vi "Module_SP_GameDisplay.vi"(8 "error in (no error)":errorcluster, 9 "Module ID":i32=-1, 10 "Wait on Module(s) (\"\": none)":string) -> (0 "error out":errorcluster)   [LabVIEW 2019, in "Module_SP_GameDisplay.lvclass"]
doc: "JSMA Module Template - SubPanels 0.2.0.9\nRob Humfeld - Jet Engineering\nCopyright (c) 2019, Jet Engineering"
uses:
  Module_SP_GameDisplay.lvclass
  <userlib>/Jet Engineering/JSMA Signal Abstraction Layer (SAL)/CORE/jModule_SAL Class/jModule_SAL_ModuleType STYP.ctl
  Private/Module_SP_GameDisplay_RxMsg STYP.ctl
  <userlib>/Jet Engineering/JSMA/Libraries/jMsg_CORE/jMsg_JSMA_ApplicationShutdown/jMsg_JSMA_ApplicationShutdown.lvclass
  C:/Program Files/National Instruments/LabVIEW 2019/user.lib/Jet Engineering/JSMA/Libraries/jMsg Class/jMsg.lvclass
  Private/Module_SP_GameDisplay_TxMsg STYP.ctl
  C:/Program Files/National Instruments/LabVIEW 2019/user.lib/Jet Engineering/JSMA GUISubPanel CORE/jModule_GUISubPanel.lvclass
  C:/Program Files/National Instruments/LabVIEW 2019/user.lib/Jet Engineering/JSMA/Libraries/jModule Class/jModule.lvclass
  C:/Program Files/National Instruments/LabVIEW 2019/user.lib/JET Engineering/JSMA Signal Abstraction Layer (SAL)/CORE/jModule_SAL Class/jModule_SAL.lvclass
  Private/Module_SP_GameDisplay_Status STYP.ctl
  <userlib>/Jet Engineering/JSMA/Libraries/jModule Class/jModule.lvclass/jModule.ctl
  Module_SP_GameDisplay.lvclass/Module_SP_GameDisplay.ctl
  <userlib>/Jet Engineering/JET_QSM/Code/Private/JET_QSM - Add State [String API].vi
  <userlib>/Jet Engineering/JET_QSM/Code/Private/JET_QSM - Add State to Front [String API].vi
  <userlib>/Jet Engineering/JSMA/Libraries/jModule Class/jModule - Set Static Timer.vi
  <userlib>/Jet Engineering/JSMA/Libraries/jModule Class/jModule - Set Periodic Timer.vi
  <vilib>/Utility/error.llb/Trim Whitespace.vi
  <vilib>/Utility/error.llb/Error Cluster From Error Code.vi
  <userlib>/Jet Labs/JET Panel/JETPanel.lvclass
  <userlib>/Jet Engineering/JSMA/Libraries/jModule Class/jModule.lvclass
  <userlib>/JET Engineering/JSMA Signal Abstraction Layer (SAL)/CORE/jModule_SAL Class/jModule_SAL.lvclass
  <userlib>/Jet Engineering/JSMA GUISubPanel CORE/jModule_GUISubPanel.lvclass
  <userlib>/Jet Engineering/JSMA Signal Abstraction Layer (SAL)/CORE/SALSignal Class/SALSignal.lvclass
panel:
  out "jModule Name":string
  out "winSizer 2":string="W"
  out "winSizer 1":string="W"
  out "Recent states before Error (with tick counts)":string="0.167 sec ago: VI Initialize\n0.167 sec ago: Window Open\n0.110 sec ago: Control Update\n0.110 sec ago: Indicator Update\n0.000 sec ago: Error Handler\r\n"
  # "CENTER"
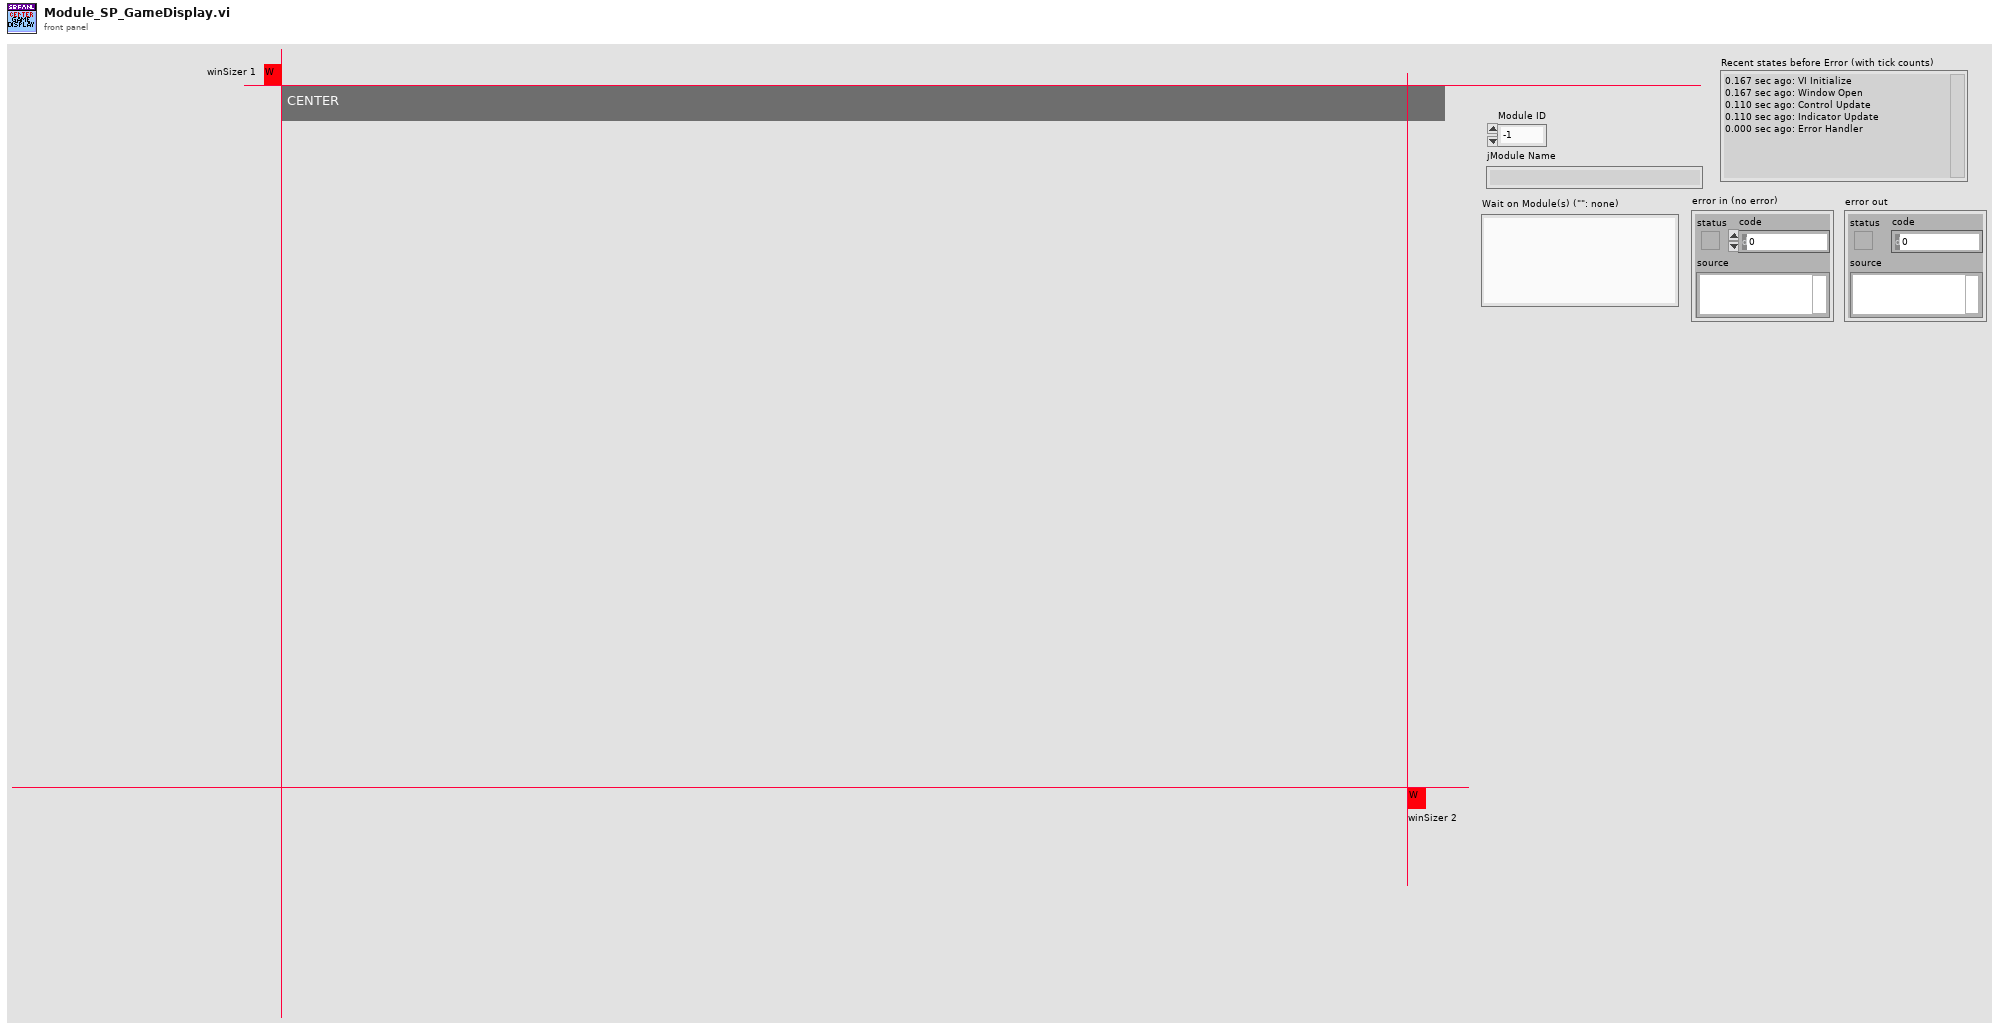
[diagram p1: front panel]
types:
  T1 = typedef "JSMA SAL CORE.lvlib/jModule_SAL.lvclass/jModule_SAL_ModuleType STYP.ctl" = enum16{"<no SAL functionality>", "Tag Data Client", "Tag Data Server", "Tag Data Server/Client"}
  T2 = typedef "Module_SP_GameDisplay.lvclass/Module_SP_GameDisplay_TxMsg STYP.ctl" = cluster{"<placeholder>":refnum<class "jMsg_JSMA_ApplicationShutdown.lvclass">}
  T3 = typedef "Module_SP_GameDisplay.lvclass/Module_SP_GameDisplay_RxMsg STYP.ctl" = cluster{"<placeholder>":refnum<class "jMsg_JSMA_ApplicationShutdown.lvclass">}
  T4 = typedef "Module_SP_GameDisplay.lvclass/Module_SP_GameDisplay_Status STYP.ctl" = cluster{"VI":cluster{"error":errorcluster, "isExiting?":bool}, "UI":cluster{"Placeholder":bool}}
  T5 = typedef "JET_QSM_Refnum STYP.ctl" = cluster{"state":cluster{"queue":refnum<queue>, "idle":string, "error":string, "STOP":string}, "debug":cluster{"enabled?":bool, "queue":refnum<queue>}, "Invalid.option":T6, "QSM.Name":string}
  T6 = typedef "JET_QSM_InvalidOption STYP.ctl" = enum16{"Ignore", "Dialog", "Error"}
  T7 = typedef "JET_QSM_Element STYP.ctl" = cluster{"state":string, "data":variant, "comment":string}
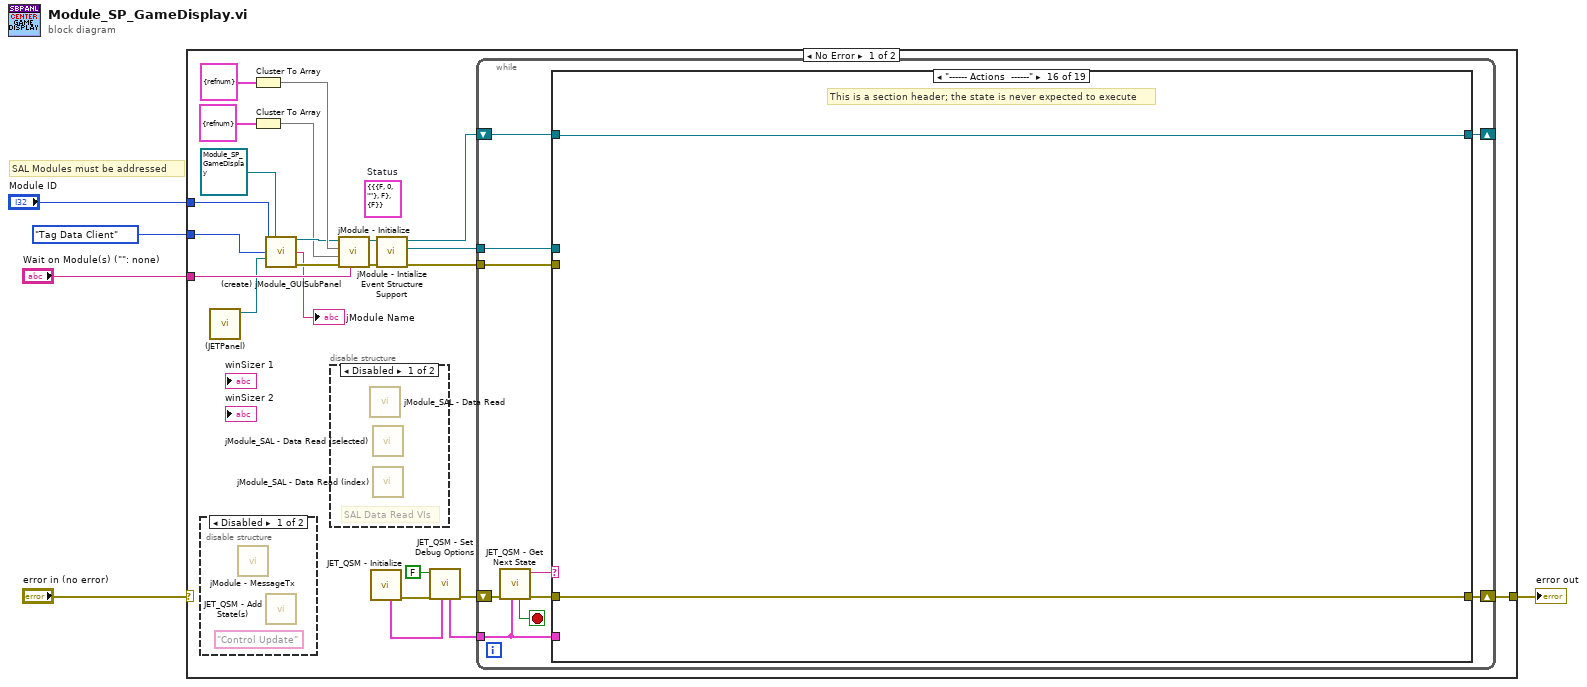
[diagram p0: block diagram]
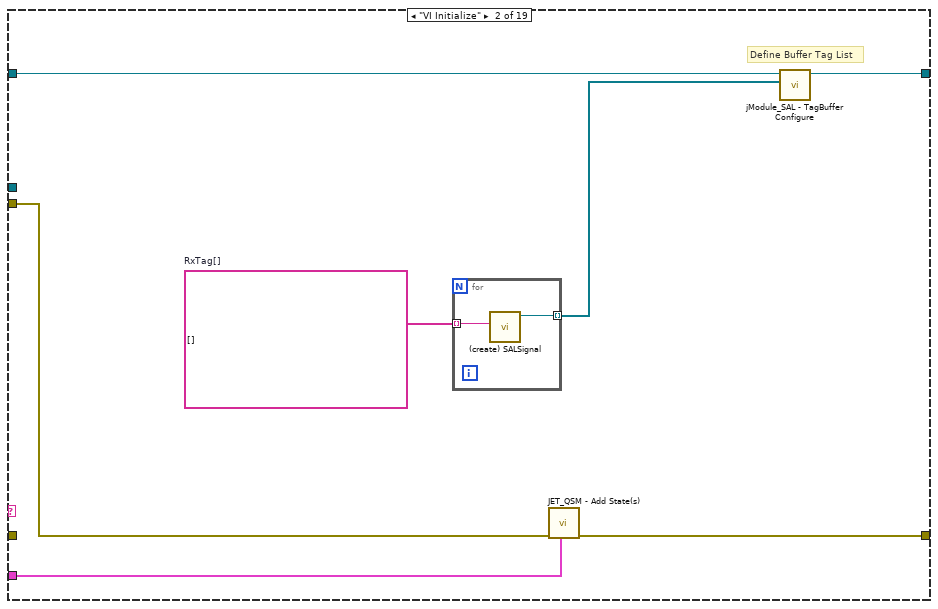
[diagram p5: hidden frame]
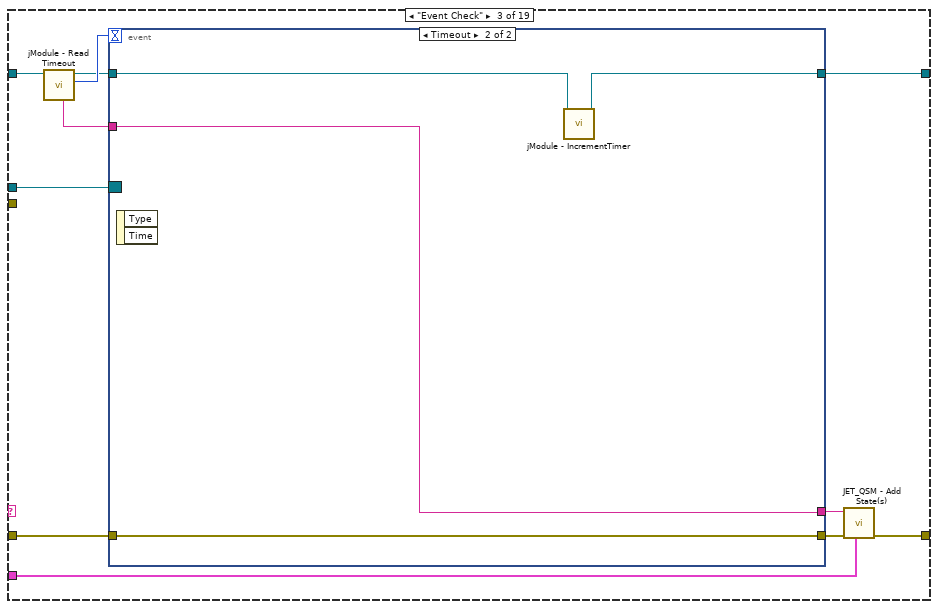
[diagram p6: hidden frame]
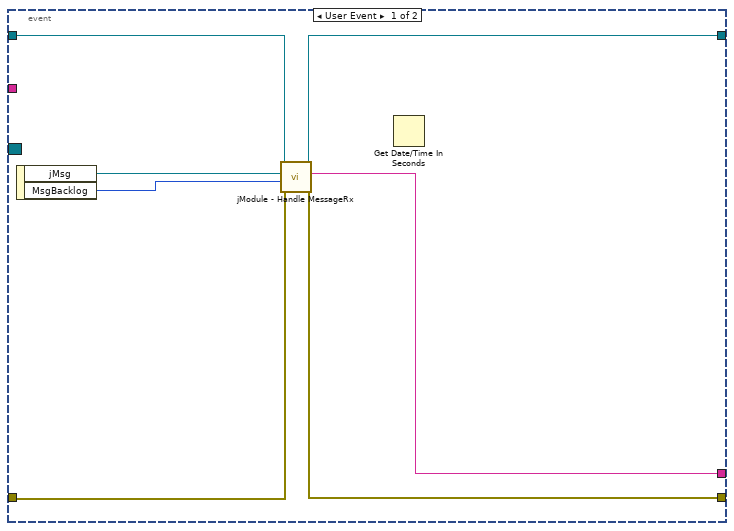
[diagram p7: hidden frame]
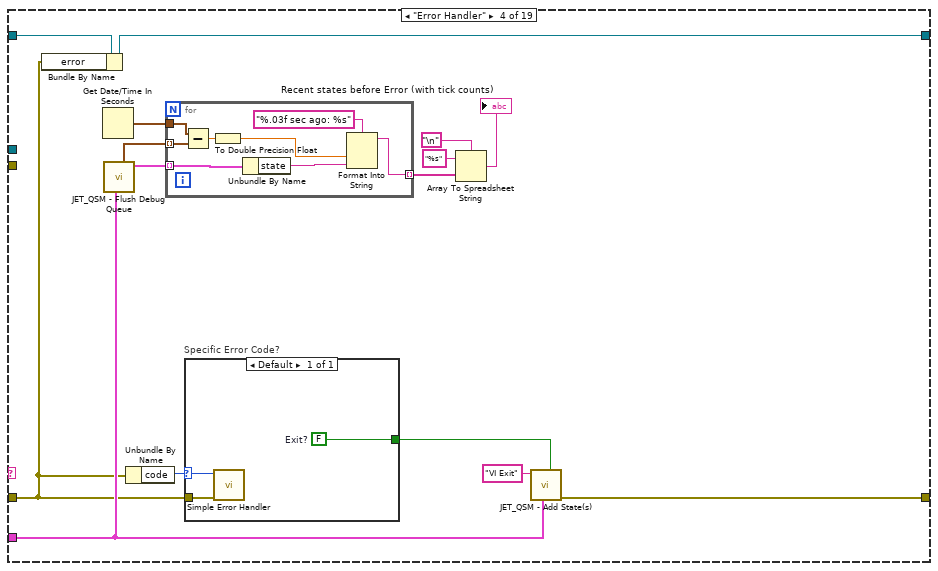
[diagram p8: hidden frame]
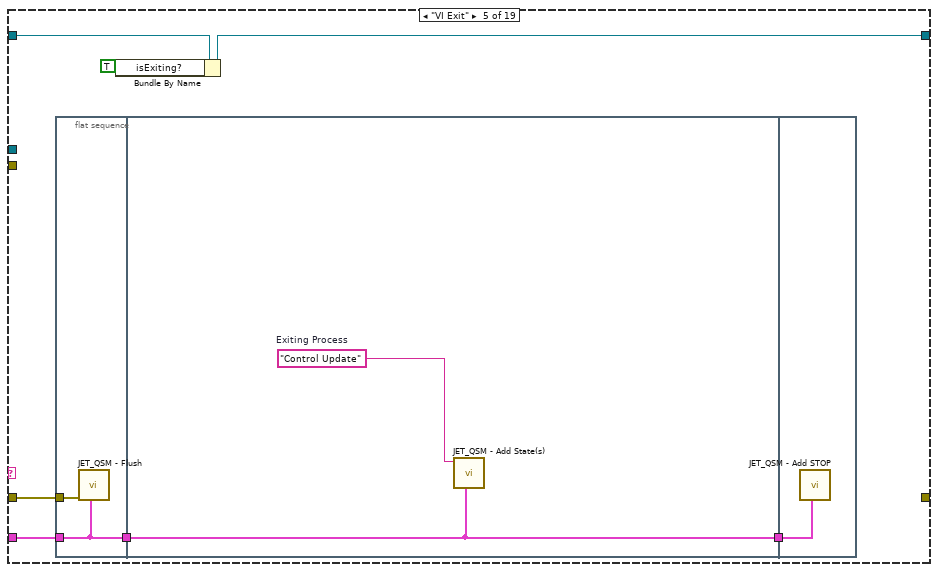
[diagram p9: hidden frame]
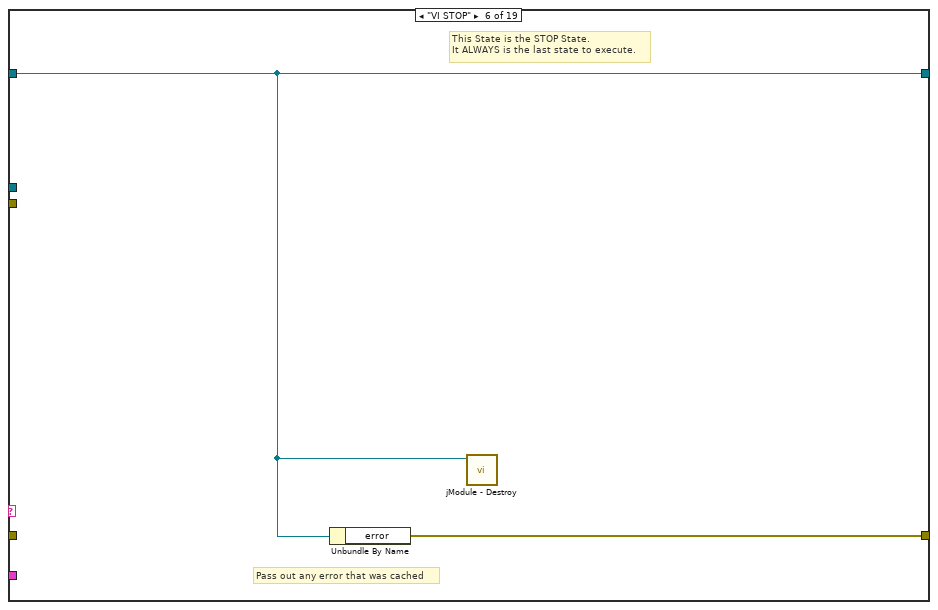
[diagram p10: hidden frame]
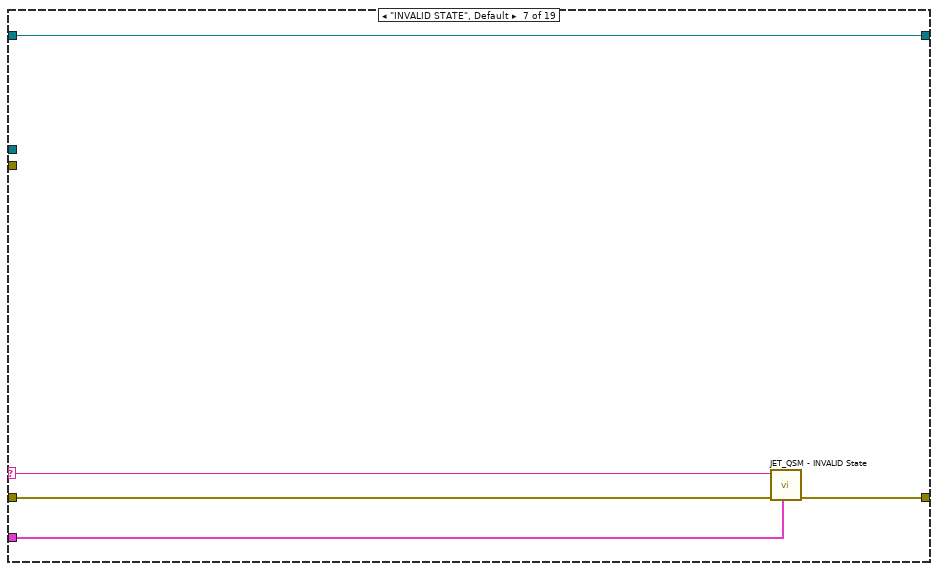
[diagram p11: hidden frame]
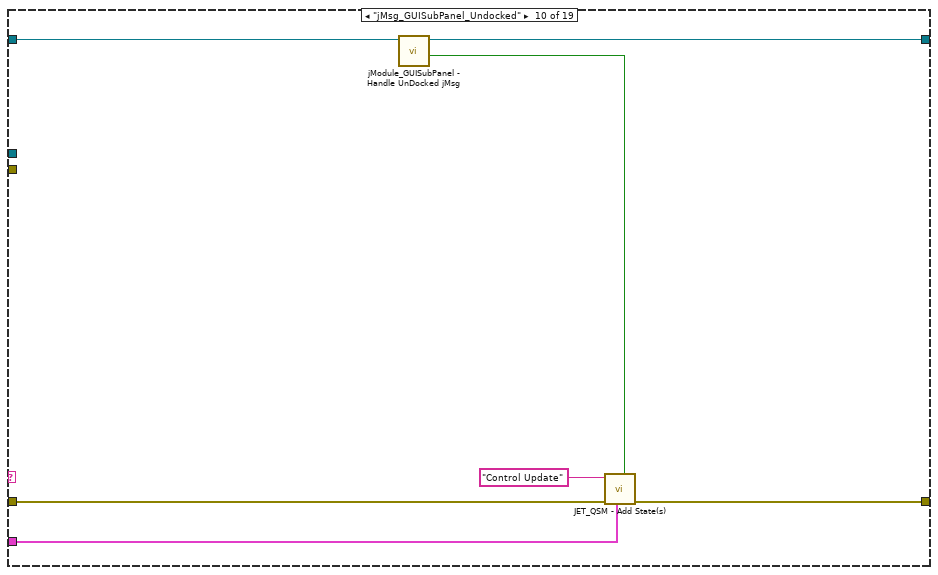
[diagram p14: hidden frame]
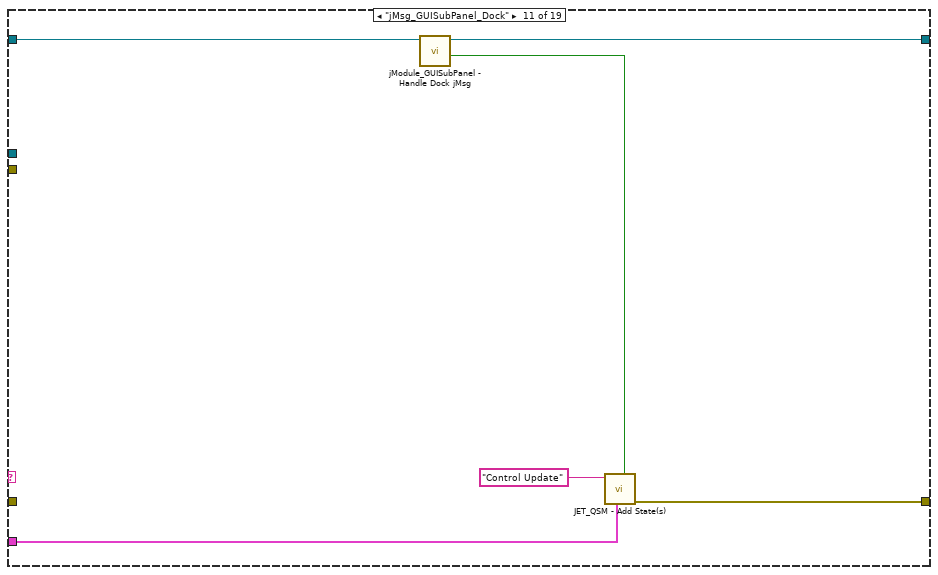
[diagram p15: hidden frame]
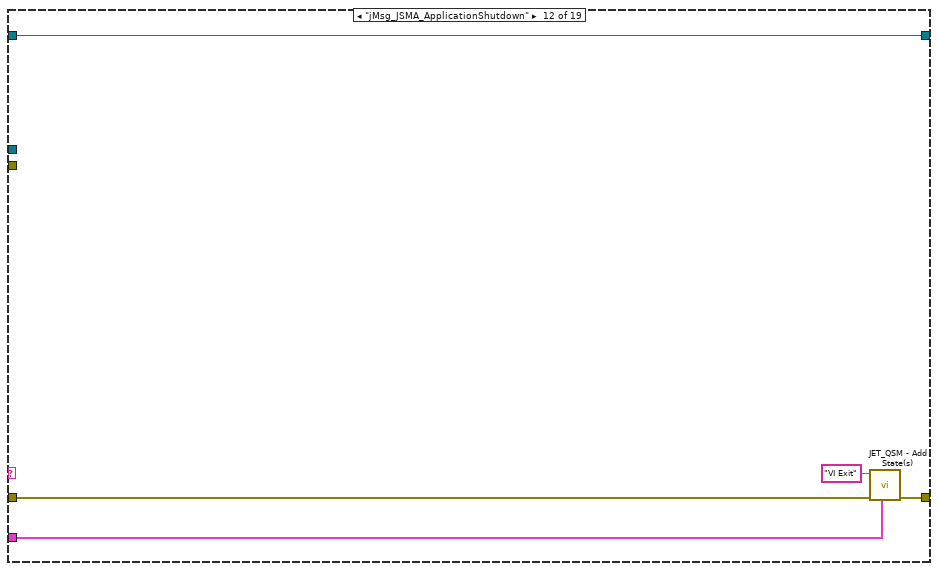
[diagram p16: hidden frame]
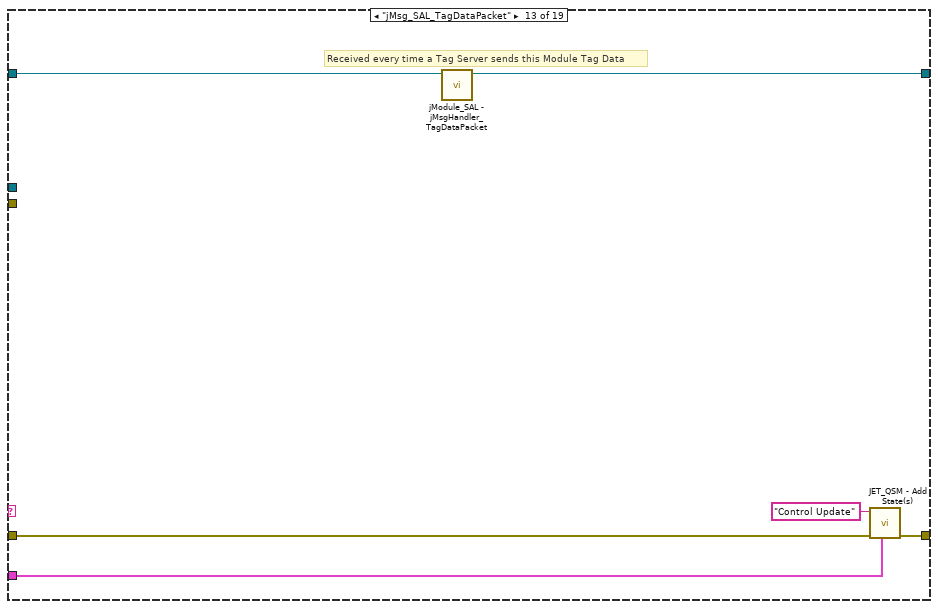
[diagram p17: hidden frame]
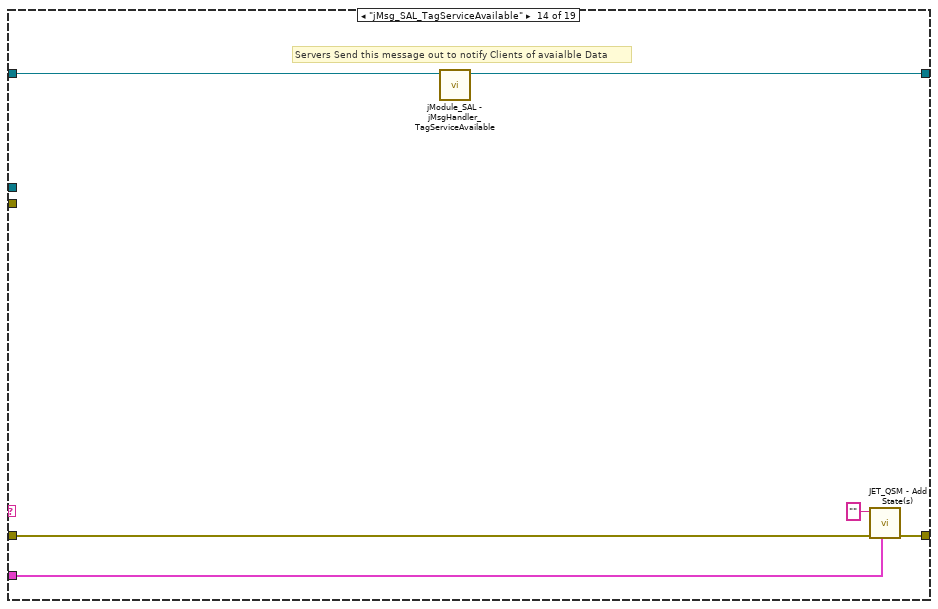
[diagram p18: hidden frame]
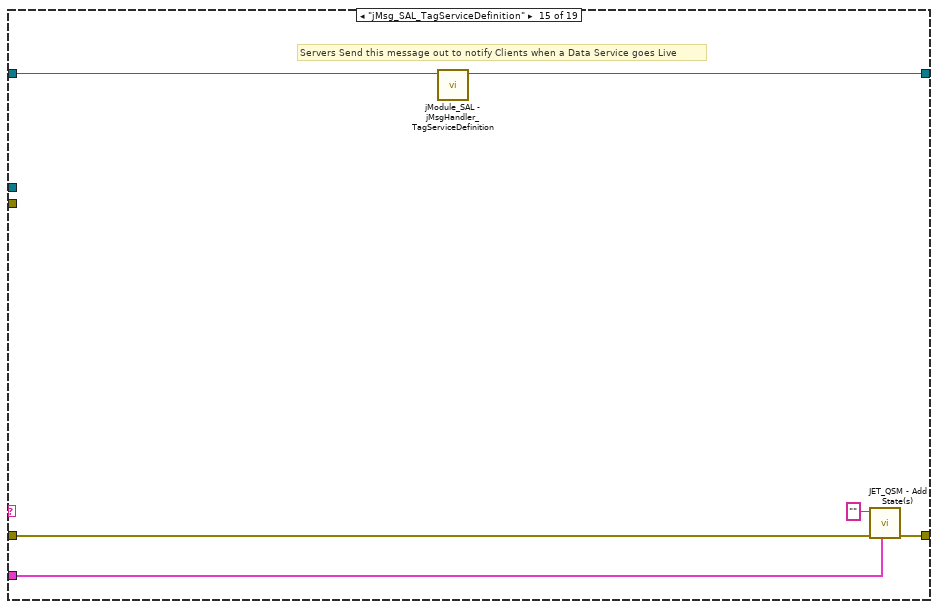
[diagram p19: hidden frame]
diagram:
  # "SAL Modules must be addressed"
  n1 = case shown="No Error" "error in (no error)" {
    selector: "error in (no error)" -> [_ w168]
    tunnel: [w28 w168] -> w5
    tunnel: "Wait on Module(s) (\"\": none)" -> [w17 _]
    tunnel: "Module ID" -> [w8 _]
    tunnel: jModule_SAL_ModuleType_STYP."Tag Data Client" ("SAL Module Type") -> [w6 _]
    frame No Error {
      (unwired) T4 {"VI"={"error"={"status"=FALSE, "code"=0, "source"=""}, "isExiting?"=FALSE}, "UI"={"Placeholder"=FALSE}}  # Status
      n2 = disable-structure shown="Disabled" {
        frame Disabled {
          (unwired) "Control Update"
          n3 = call <userlib>:"jModule - MessageTx.vi"() -> ()  [unwired: 8 in, 4 out]
          n4 = call-poly <userlib>:"JET_QSM - Add State(s).vi"() -> ()  [unwired: 11 in, 1 out]
        }
        frame Enabled {
        }
      }
      n5 = call <userlib>:"(JETPanel).vi"() -> ("JETPanel"=w10:refnum<class "JETPanel.lvclass">)  [unwired: 8 in, 3 out]
      n6 = Cluster To Array(cluster=T2 {"<placeholder>"=refnum} ("TxMsg")) -> (array=w22:refnum<class "jMsg_JSMA_ApplicationShutdown.lvclass">[])
      n7 = Cluster To Array(cluster=T3 {"<placeholder>"=refnum} ("RxMsg")) -> (array=w9:refnum<class "jMsg_JSMA_ApplicationShutdown.lvclass">[])
      n8 = call <userlib>:"(create) jModule_GUISubPanel.vi"("jModule_GUISubPanel child class"=refnum<class "Module_SP_GameDisplay.lvclass"> refnum ("Module_UI_SystemEventLog.lvclass"), "Module ID"=w8, "SAL Module Type"=w6, "JETPanel"=w10) -> ("jModule_GUISubPanel"=w12:refnum<class "Module_SP_GameDisplay.lvclass">, "jModule Name"=→"jModule Name":string, "error out"=w11:errorcluster)  [unwired: 8 in, 1 out]
      n9 = disable-structure shown="Disabled" {
        frame Disabled {
          # "SAL Data Read VIs"
          n10 = call-dynamic "jModule_SAL - Data Read.vi"() -> ()  [unwired: 8 in, 4 out]
          n11 = call-dynamic "jModule_SAL - Data Read (selected).vi"() -> ()  [unwired: 9 in, 3 out]
          n12 = call-dynamic "jModule_SAL - Data Read (index).vi"() -> ()  [unwired: 9 in, 3 out]
        }
        frame Enabled {
        }
      }
      n13 = call-dynamic "jModule - Initialize.vi"("Wait on Module(s) (\"\": none)"=w17, "error in (no error)"=w11, "jMsgRxList"=w9, "jMsgTxList"=w22, "jModule Template_SubPanel UI (Center)"=w12) -> ("error out"=w21:errorcluster, "jModule Template_SubPanel UI (Center)"=w20:refnum<class "Module_SP_GameDisplay.lvclass">)  [unwired: 5 in]
      n14 = call <userlib>:"JET_QSM - Initialize.vi"() -> ("error out"=w23:errorcluster, "Jet_QSM refnum"=w26:T5)  [unwired: 10 in]
      n15 = call <userlib>:"jModule - Intialize Event Structure Support.vi"("error in (no error)"=w21, "jModule"=w20) -> ("error out"=w18:errorcluster, "Event Registration Refnum"=w19:refnum<event-registration>, "jModule"=w14:refnum<class "Module_SP_GameDisplay.lvclass">)  [unwired: 6 in, 1 out]
      n16 = call <userlib>:"JET_QSM - Set Debug Options.vi"("Jet_QSM refnum"=w26, "error in (no error)"=w23, "debug.enabled? (F)"=FALSE) -> ("error out"=w24:errorcluster, "Jet_QSM ref"=w25:T5)  [unwired: 7 in]
      n17 = while {
        tunnel: w25 -> [w34]
        shift-right: [w32] -> _
        shift-left: w14 -> [w33]
        shift-right: [w31] -> w28
        shift-left: w24 -> [w38]
        tunnel: w18 -> [w30]
        tunnel: w19 -> [w29]
        stop <- w35 stop-if-true
        n18 = call <userlib>:"JET_QSM - Get Next State.vi"("Jet_QSM refnum"=w34, "error in (no error)"=w38) -> ("error out"=w37:errorcluster, "state"=w36:string, "Stop Loop?"=w35:bool)  [unwired: 5 in, 2 out]
        n19 = case shown="\"------ Actions  ------\"" w36 {
          selector: w36 -> [_ _ _ _ _ _ w112 _ _ _ _ _ _ _ _ _ _ _ _]
          tunnel: w37 -> [w39 _ w60 w74 w104 _ w114 w117 w119 w121 _ w134 w141 w147 w153 w157 w159 w164 w167]
          tunnel: w34 -> [_ w47 w59 w78 w103 _ w115 _ _ w127 w133 w138 w144 w150 w156 _ _ w165 _]
          tunnel: w33 -> [w40 w44 w51 w73 w101 w110 w113 w118 w120 w124 w130 w135 w140 w146 w152 w158 w160 w161 w166]
          tunnel: [w40 w43 w55 w72 w100 w110 w113 w118 w120 w123 w129 w135 w139 w145 w151 w158 w160 w161 w166] -> w32
          tunnel: [w39 w46 w57 w79 _ w111 w116 w117 w119 w126 w132 w137 w143 w149 w155 w157 w159 w163 w167] -> w31
          tunnel: w30 -> [_ w45 _ _ _ _ _ _ _ _ _ _ _ _ _ _ _ _ _]
          tunnel: w29 -> [_ _ w54 _ _ _ _ _ _ _ _ _ _ _ _ _ _ _ _]
          frame "------ Standard States ------" {
            # "Standard States are required states for a JET_QSM State Machine\n\nTheir names may be changed; use the Initialize function to specify the new names"
            # "This is a section header; the state is never expected to execute"
          }
          frame "VI Initialize" {
            w42 = string[] []  # RxTag[]
            # "Define Buffer Tag List"
            n20 = for {
              tunnel: w42 -> [w49] mode=indexing
              tunnel: [w48] -> w41 mode=indexing
              n21 = call <userlib>:"(create) SALSignal.vi"("Tag"=w49) -> ("SALSignal"=w48:refnum<class "SALSignal.lvclass">)  [unwired: 9 in, 1 out]
            }
            n22 = call-poly <userlib>:"JET_QSM - Add State(s).vi"("Jet_QSM refnum"=w47, "error in (no error)"=w45) -> ("error out"=w46:errorcluster)  [unwired: 9 in]
            n23 = call <userlib>:"jModule_SAL - TagBuffer Configure.vi"("Server.SALSignal[]"=w41, "jModule_SAL"=w44) -> ("jModule_SAL"=w43:refnum<class "Module_SP_GameDisplay.lvclass">)  [unwired: 7 in, 2 out]
          }
          frame "Event Check" {
            n24 = call <userlib>:"jModule - Read Timeout.vi"("jModule"=w51) -> ("Timeout, ms"=w53:i32, "jModule"=w50:refnum<class "Module_SP_GameDisplay.lvclass">, "Timeout.State"=w52:string)  [unwired: 8 in]
            n25 = event shown="[1] Timeout" {
              selector: w54 -> [_ _]
              dyn-events: _ -> [_ _]
              timeout: w53 -> [_ _]
              tunnel: w60 -> [w65 w70]
              tunnel: [w66 w71] -> w58
              tunnel: [w64 w70] -> w56
              tunnel: w50 -> [w62 w69]
              tunnel: [w61 w68] -> w55
              tunnel: w52 -> [_ w71]
              event User Event {
                n26 = event-data() -> ("jMsg"=w67:refnum<class "jMsg.lvclass">, "MsgBacklog"=w63:i32)  [unwired: 1 in]
                n27 = call-dynamic "jModule - Handle MessageRx.vi"("error in (no error)"=w65, "Message Backlog"=w63, "jMsg"=w67, "jModule"=w62) -> ("error out"=w64:errorcluster, "QSMState"=w66:string, "jModule"=w61:refnum<class "Module_SP_GameDisplay.lvclass">)  [unwired: 4 in, 1 out]
                n28 = Get Date/Time In Seconds() -> ()  [unwired: 1 out]
              }
              event Timeout {
                n29 = event-data() -> ()  [unwired: 1 in, 2 out]
                n30 = call <userlib>:"jModule - IncrementTimer.vi"("jModule"=w69) -> ("jModule"=w68:refnum<class "Module_SP_GameDisplay.lvclass">)  [unwired: 10 in]
              }
            }
            n31 = call-poly <userlib>:"JET_QSM - Add State(s).vi"("Jet_QSM refnum"=w59, "error in (no error)"=w56, "state(s)"=w58) -> ("error out"=w57:errorcluster)  [unwired: 8 in]
          }
          frame "Error Handler" {
            n32 = Bundle By Name(cluster=w73, "error"=w74) -> (w72:refnum<class "Module_SP_GameDisplay.lvclass">)
            n33 = Get Date/Time In Seconds() -> (seconds since 1Jan1904=w82:timestamp)
            n34 = call <userlib>:"JET_QSM - Flush Debug Queue.vi"("Jet_QSM refnum"=w78) -> ("QSM Elements"=w80:T7[], "Timestamps"=w81:timestamp[])  [unwired: 8 in, 1 out]
            n35 = Unbundle By Name(w74) -> ("code"=w75:i32)
            n36 = for {
              tunnel: w80 -> [w94] mode=indexing
              tunnel: [w92] -> w84 mode=indexing
              tunnel: w82 -> [w89]
              tunnel: w81 -> [w90] mode=indexing
              n37 = Subtract(x=w89, y=w90) -> (x-y=w88:dbl)
              n38 = To Double Precision Float(number=w88) -> (double precision float=w87:dbl)
              n39 = Unbundle By Name(w94) -> ("state"=w93:string)
              n40 = Format Into String(format string="%.03f sec ago: %s", w87, w93) -> (resulting string=w92:string)  [unwired: 2 in, 1 out]
            }
            n41 = case "Specific Error Code?" shown="Default" w75 {
              selector: w75 -> [w96]
              tunnel: [w97] -> w76
              tunnel: w74 -> [w95]
              frame Default {
                w97 = FALSE  # Exit?
                n42 = call <vilib>:"Simple Error Handler.vi"("error code (no error:0)"=w96, "error in (no error)"=w95) -> ()  [unwired: 3 in, 5 out]
              }
            }
            n43 = Array To Spreadsheet String(delimiter (Tab)="\n", array=w84, 3:"%s" ("format string")) -> (spreadsheet string=→"Recent states before Error (with tick counts)":string)
            n44 = call-poly <userlib>:"JET_QSM - Add State(s).vi"("act? (T)"=w76, "Jet_QSM refnum"=w78, "state(s)"="VI Exit") -> ("error out"=w79:errorcluster)  [unwired: 8 in]
          }
          frame "VI Exit" {
            n45 = flat-sequence {
              tunnel: w104 -> [w106]
              tunnel: w103 -> [w105]
              tunnel: [w105] -> w102
              tunnel: w102 -> [w108]
              tunnel: [w108] -> w98
              tunnel: w98 -> [w109]
              frame #0 {
                n46 = call <userlib>:"JET_QSM - Flush.vi"("Jet_QSM ref"=w105, "error in (no error)"=w106) -> ()  [unwired: 8 in, 2 out]
              }
              frame #1 {
                w107 = "Control Update"  # Exiting Process
                n47 = call-poly <userlib>:"JET_QSM - Add State(s).vi"("Jet_QSM refnum"=w108, "state(s)"=w107) -> ()  [unwired: 9 in, 1 out]
              }
              frame #2 {
                n48 = call <userlib>:"JET_QSM - Add STOP.vi"("Jet_QSM refnum"=w109) -> ()  [unwired: 10 in, 1 out]
              }
            }
            n49 = Bundle By Name(cluster=w101, "isExiting?"=TRUE ("VI.isExiting?")) -> (w100:refnum<class "Module_SP_GameDisplay.lvclass">)
          }
          frame "VI STOP" {
            # "Pass out any error that was cached"
            # "This State is the STOP State.\nIt ALWAYS is the last state to execute."
            n50 = Unbundle By Name(w110) -> ("error"=w111:errorcluster)
            n51 = call-dynamic "jModule - Destroy.vi"("jModule_GUISubPanel"=w110) -> ()  [unwired: 10 in, 1 out]
          }
          frame "INVALID STATE", Default {
            n52 = call <userlib>:"JET_QSM - INVALID State.vi"("Jet_QSM refnum"=w115, "error in (no error)"=w114, "state"=w112) -> ("error out"=w116:errorcluster)  [unwired: 8 in]
          }
          frame "------ Menu Commands ------" {
            # "This is a section header; the state is never expected to execute"
          }
          frame "------ jMsg  ------" {
            # "This is a section header; the state is never expected to execute"
          }
          frame "jMsg_GUISubPanel_Undocked" {
            n53 = call-dynamic "jModule_GUISubPanel - Handle UnDocked jMsg.vi"("jModule_GUISubPanel"=w124) -> ("Undocked?"=w122:bool, "jModule_GUISubPanel"=w123:refnum<class "Module_SP_GameDisplay.lvclass">)  [unwired: 7 in, 2 out]
            n54 = call-poly <userlib>:"JET_QSM - Add State(s).vi"("act? (T)"=w122, "Jet_QSM refnum"=w127, "error in (no error)"=w121, "state(s)"="Control Update") -> ("error out"=w126:errorcluster)  [unwired: 7 in]
          }
          frame "jMsg_GUISubPanel_Dock" {
            n55 = call-dynamic "jModule_GUISubPanel - Handle Dock jMsg.vi"("jModule_GUISubPanel"=w130) -> ("Docked?"=w128:bool, "jModule_GUISubPanel"=w129:refnum<class "Module_SP_GameDisplay.lvclass">)  [unwired: 5 in, 4 out]
            n56 = call-poly <userlib>:"JET_QSM - Add State(s).vi"("act? (T)"=w128, "Jet_QSM refnum"=w133, "state(s)"="Control Update") -> ("error out"=w132:errorcluster)  [unwired: 8 in]
          }
          frame "jMsg_JSMA_ApplicationShutdown" {
            n57 = call-poly <userlib>:"JET_QSM - Add State(s).vi"("Jet_QSM refnum"=w138, "error in (no error)"=w134, "state(s)"="VI Exit") -> ("error out"=w137:errorcluster)  [unwired: 8 in]
          }
          frame "jMsg_SAL_TagDataPacket" {
            # "Received every time a Tag Server sends this Module Tag Data"
            n58 = call-dynamic "jModule_SAL - jMsgHandler_TagDataPacket.vi"("jModule_SAL"=w140) -> ("jModule_SAL"=w139:refnum<class "Module_SP_GameDisplay.lvclass">)  [unwired: 3 in, 7 out]
            n59 = call-poly <userlib>:"JET_QSM - Add State(s).vi"("Jet_QSM refnum"=w144, "error in (no error)"=w141, "state(s)"="Control Update") -> ("error out"=w143:errorcluster)  [unwired: 8 in]
          }
          frame "jMsg_SAL_TagServiceAvailable" {
            # "Servers Send this message out to notify Clients of avaialble Data"
            n60 = call-dynamic "jModule_SAL - jMsgHandler_TagServiceAvailable.vi"("jModule_SAL"=w146) -> ("jModule_SAL"=w145:refnum<class "Module_SP_GameDisplay.lvclass">)  [unwired: 4 in, 6 out]
            n61 = call-poly <userlib>:"JET_QSM - Add State(s).vi"("Jet_QSM refnum"=w150, "error in (no error)"=w147, "state(s)"="") -> ("error out"=w149:errorcluster)  [unwired: 8 in]
          }
          frame "jMsg_SAL_TagServiceDefinition" {
            # "Servers Send this message out to notify Clients when a Data Service goes Live"
            n62 = call <userlib>:"jModule_SAL - jMsgHandler_TagServiceDefinition.vi"("jModule_SAL"=w152) -> ("jModule_SAL"=w151:refnum<class "Module_SP_GameDisplay.lvclass">)  [unwired: 3 in, 7 out]
            n63 = call-poly <userlib>:"JET_QSM - Add State(s).vi"("Jet_QSM refnum"=w156, "error in (no error)"=w153, "state(s)"="") -> ("error out"=w155:errorcluster)  [unwired: 8 in]
          }
          frame "------ Actions  ------" {
            # "This is a section header; the state is never expected to execute"
          }
          frame "------ Window and Panel Control ------" {
            # "This is a section header; the state is never expected to execute"
          }
          frame "Control Update" {
            # "Update all control properties here from the status cluster\n(Consolidate/reduce property nodes)"
            n64 = call-poly <userlib>:"JET_QSM - Add State(s).vi"("Jet_QSM refnum"=w165, "error in (no error)"=w164, "state(s)"="Indicator Update") -> ("error out"=w163:errorcluster)  [unwired: 8 in]
          }
          frame "Indicator Update" {
            # "Update all indicator values here from the status cluster\n(Eliminate Local Variables)"
          }
        }
      }
    }
    frame Error {
    }
  }
  "error out" <- w5
